vi "Set Stream State Register.vi"(7 "stream state register":T2, 10 "stream.state":T1) -> (6 "ready for input":bool)   [LabVIEW 2015, in "niInstr Streaming v1 FPGA.lvlib"]
uses:
  <instrlib>/_niInstr/Streaming/v1/FPGA/niInstr Streaming v1 FPGA.lvlib
  <instrlib>/_niInstr/Streaming/v1/FPGA/Public/Stream State Register.ctl
  <instrlib>/_niInstr/Streaming/v1/Common/Stream State.ctl
  <vilib>/rvi/Emulation/niFpgaSctlEmulationGetInTimedLoop.vi
  <vilib>/Utility/error.llb/Clear Errors.vi
  <vilib>/rvi/DataTransferAndStorage/Container/Common/niFpgaContainerGetUniqueNameForEmu.vi
  <vilib>/rvi/DataTransferAndStorage/Container/Common/niFpgaContainerSetEmuInfo.vi
  <vilib>/rvi/eio/common/nirviEmuReportErrorAndStop.vi
  <vilib>/rvi/DataTransferAndStorage/Container/Common/niFpgaContainerExecOnDevCompGetState.vi
  <vilib>/rvi/Emulation/niFpgaEmulationIsFPGAContextNoSignature.vi
  <vilib>/rvi/errors/niFpgaSetErrorForExecOnDevCompSimple.vi
  <vilib>/rvi/FIFO/Fifo_Resource/nirvififoEmulationSetSize.vi
  <vilib>/rvi/FIFO/Fifo_Resource/nirviFifoEmulationQueueMgr.vi
  <instcachedir>/0/nirviFifoEmulationQueueMgr_E5CAEC123FF24DC58D834DCA3CDAA9B5.lvgen/nirviFifoEmulationQueueMgr_E5CAEC123FF24DC58D834DCA3CDAA9B5_009.vi
  <vilib>/rvi/FIFO/Fifo_Resource/nirvififoEmulationDetermineInputValidOut.vi
  <vilib>/rvi/FIFO/Fifo_Resource/nirvififoEmulationCreateLock.vi
  <vilib>/rvi/Emulation/niFpgaProcessEmulError.vi
  <vilib>/rvi/FIFO/Fifo_Resource/nirvififoEmulationObtainLock.vi
  <vilib>/rvi/FIFO/Fifo_Resource/nirvififoEmulationReleaseLock.vi
  <vilib>/rvi/occurrence/nirviWaitOnOccurrenceBase.vi
  <vilib>/rvi/errors/nirviReportUnexpectedCaseInternalError.vi
  <vilib>/rvi/errors/nirviReportUnexpectedCaseInternalError (U32).vi
  <vilib>/rvi/interface/RandomDataEmulation/niFpgaRandomDataHandleErrors.vi
  <vilib>/rvi/LocalResourceManager/LocalResourceManager.xnode
  <vilib>/rvi/DataTransferAndStorage/Container/XNode/niFpgaContainer.xnode
  <vilib>/rvi/FIFO/Fifo_Resource/niFpgaFifoEmulationRefIn.vi
  <vilib>/rvi/DataTransferAndStorage/Handshake/Emulation/niFpgaHandshakeEmulationRefIn.vi
  <instrlib>/_niInstr/Streaming/v1/Common/niInstr Streaming v1 Common.lvlib
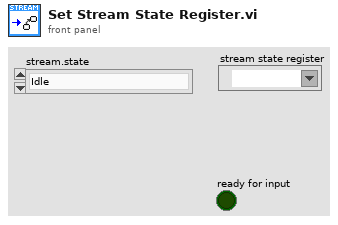
[diagram p1: front panel]
types:
  T1 = typedef "niInstr Streaming v1 Common.lvlib/Stream State.ctl" = enum8{"Idle", "Finite Transfer", "Continuous", "Done", "Error", "Not Ready", "Cancel"}
  T2 = typedef "niInstr Streaming v1 FPGA.lvlib/Stream State Register.ctl" = refnum<k21>
  T3 = enum8{"Idle", "Finite Transfer", "Continuous", "Done", "Error", "Not Ready", "Cancel"}
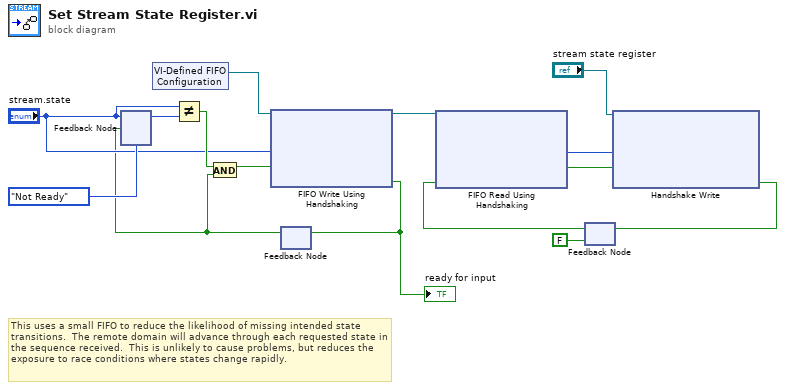
[diagram p0: block diagram]
diagram:
  # "This uses a small FIFO to reduce the likelihood of missing intended state transitions.  The remote domain will advance through each requested state in the sequence received.  This is unlikely to cause problems, but reduces the exposure to race conditions where states change rapidly."
  n1 = feedback #1(Stream_State."Not Ready" ("stream.state")) -> (w13:T1)
  n2 = xnode "VI-Defined FIFO Configuration"() -> ("FIFO Out"=w11:refnum<k21>)
  n3 = Not Equal?(x="stream.state", y=w13) -> (x != y?=w10:bool)
  n4 = feedback #2() -> (w1:bool)  [unwired: 1 in]
  n5 = feedback-in #1("stream.state", w1) -> ()
  n6 = And(x=w10, y=w1) -> (x .and. y?=w2:bool)
  n7 = xnode ("FIFO Write Using Handshaking")("Element"="stream.state", "Input Valid"=w2, "FIFO In"=w11) -> ("Ready for Input"=w3:bool, "FIFO Out"=w8:refnum<k21>)
  "ready for input" <- w3
  n8 = feedback-in #2(w3) -> ()
  n9 = feedback #3(FALSE ("Ready for Input")) -> (w5:bool)
  n10 = xnode ("FIFO Read Using Handshaking")("Ready for Output"=w5, "FIFO In"=w8) -> ("Element"=w7:T3, "Output Valid"=w6:bool)  [unwired: 1 out]
  n11 = xnode ("Handshake Write")("Data"=w7, "Input Valid"=w6, "Handshake In"="stream state register") -> ("Ready for Input"=w14:bool)  [unwired: 1 out]
  n12 = feedback-in #3(w14) -> ()
